vi "Get Settings File path from Command Params.vi"(8 "error in (no error)":errorcluster, 11 "Params Array IN":string[][](array[string])) -> (0 "error out":errorcluster, 3 "Settings Path OUT":path)   [LabVIEW 2012]
doc: "SciScan 1.2 160622"
uses:
  SubVIs/MacroFileIO_Commands.ctl
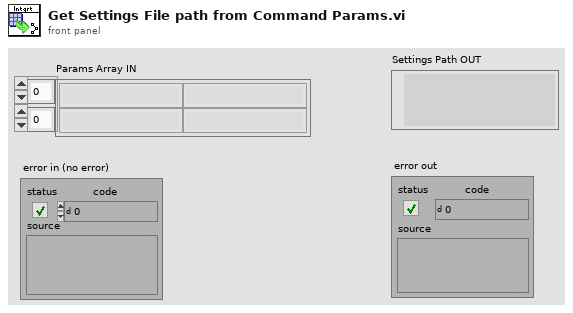
[diagram p1: front panel]
types:
  T1 = typedef "MacroFileIO_Commands.ctl" = enum16{"Get Macro Info", "Initialize", "New Macro", "Load Macro", "Save", "Save in today's folder", "Update Settings File", "Add Settings File", "Delete Settings File", "Update Macro Text", "Save As", "Read Temp File"}
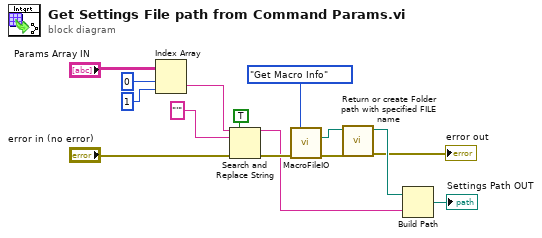
[diagram p0: block diagram]
diagram:
  n1 = Index Array(array="Params Array IN", index (row)=0, index (col)=1 ("disabled index (col)")) -> (element=w12:string)
  n2 = Search and Replace String(replace all?=TRUE ("replace all? (F)"), input string=w12, search string="'", error in="error in (no error)") -> (result string=w10:string, error out=w11:errorcluster)  [unwired: 4 in, 2 out]
  n3 = call "MacroFileIO.vi"("MacroFileIO_Command"=MacroFileIO_Commands."Get Macro Info", "Error In"=w11) -> ("Temp File path"=w7:path, "Error Out"=w8:errorcluster)  [unwired: 8 in, 4 out]
  n4 = call "Return or create Folder path with specified FILE name.vi"("error in (no error)"=w8, "File Path IN"=w7) -> ("error out"=→"error out":errorcluster, "Folder Path OUT"=w6:path)  [unwired: 8 in]
  n5 = Build Path(base path=w6, name or relative path=w10) -> (appended path=→"Settings Path OUT":path)
